vi "Prepend Test Project Path If New.vi"(8 "error in":errorcluster, 11 "Test Project":path) -> (0 "error out":errorcluster)   [LabVIEW 2013, in "GraphicalTestRunner.lvlib"]
uses:
  GraphicalTestRunner.lvlib
  <userlib>/_OpenG.lib/array/array.llb/Filter 1D Array with Scalar (Path)__ogtk.vi
  <userlib>/_OpenG.lib/array/array.llb/Filter 1D Array (Path)__ogtk.vi
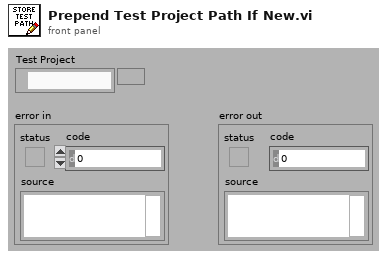
[diagram p1: front panel]
types:
  T1 = cluster{"Recent Paths":path[], "SkipMassCompileCheck":bool}
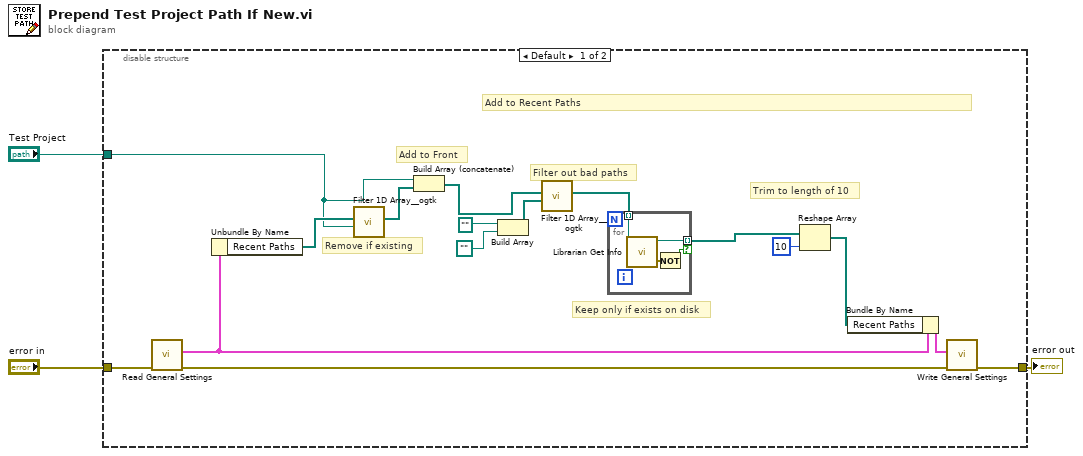
[diagram p0: block diagram]
diagram:
  n1 = disable-structure shown="Default" {
    disable-tunnel: [w19 w24] -> w3
    disable-tunnel: "error in" -> [w18 w24]
    disable-tunnel: "Test Project" -> [w15 _]
    frame condition #0 (active) {
      # "Keep only if exists on disk"
      # "Filter out bad paths"
      # "Trim to length of 10"
      # "Add to Front"
      # "Remove if existing"
      # "Add to Recent Paths"
      n2 = call "Read General Settings.vi"("error in"=w18) -> ("error out"=w17:errorcluster, "General"=w14:T1)  [unwired: 9 in]
      n3 = Unbundle By Name(w14) -> ("Recent Paths"=w16:path[])
      n4 = call-poly <userlib>:"Filter 1D Array__ogtk.vi"("items to filter"=w15, "array"=w16) -> ("filtered array"=w8:path[])  [unwired: 4 in, 1 out]
      n5 = Build Array (concatenate)(w15, w8) -> (w7:path[])
      n6 = Build Array(path "", path "") -> (w9:path[])
      n7 = call-poly <userlib>:"Filter 1D Array__ogtk.vi"("items to filter"=w9, "array"=w7) -> ("filtered array"=w5:path[])  [unwired: 4 in, 1 out]
      n8 = for {
        tunnel: w5 -> [w23] mode=indexing
        tunnel: [w22] -> w4 mode=indexing if=w20
        n9 = call <vilib>:"Librarian Get Info.vi"("path"=w23) -> ("error out"=w21:errorcluster, "dup path"=w22:path)  [unwired: 8 in, 1 out]
        n10 = Not(x=w21) -> (.not. x?=w20:bool)
      }
      n11 = Reshape Array(w4, 10 ("dimension size")) -> (w6:path[])
      n12 = Bundle By Name(cluster=w14, "Recent Paths"=w6) -> (w12:T1)
      n13 = call "Write General Settings.vi"("error in"=w17, "General"=w12) -> ("error out"=w19:errorcluster)  [unwired: 9 in]
    }
    frame condition #1 {
      # "don't save path if in a built EXE"
    }
  }
  "error out" <- w3
